vi "GFITS_HdrType2.vi"(10 "keyval":string) -> (1 "type":string, 2 "keyval out":string, 3 "specified":bool)   [LabVIEW 2016]
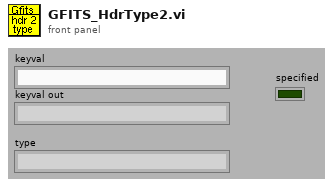
[diagram p1: front panel]
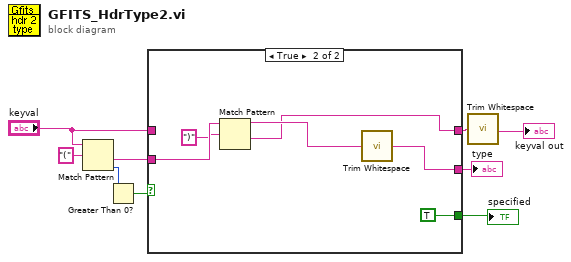
[diagram p0: block diagram]
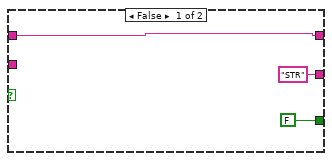
[diagram p2: hidden frame]
diagram:
  n1 = Match Pattern(string="keyval", regular expression="(") -> (after substring=w8:string, offset past match=w7:i32)  [unwired: 3 out]
  n2 = Greater Than 0?(x=w7) -> (x > 0?=w6:bool)
  n3 = case shown="True" w6 {
    tunnel: w8 -> [_ w18]
    tunnel: "keyval" -> [w12 _]
    tunnel: [w12 w14] -> w4
    tunnel: ["STR" ("trimmed string") w16] -> w3
    tunnel: [FALSE ("specified") TRUE ("specified")] -> w1
    frame False {
    }
    frame True {
      n4 = Match Pattern(string=w18, regular expression=")") -> (before substring=w15:string, after substring=w14:string)  [unwired: 3 out]
      n5 = call <vilib>:"Trim Whitespace.vi"("string"=w15) -> ("trimmed string"=w16:string)  [unwired: 1 in]
    }
  }
  "type" <- w3
  "specified" <- w1
  n6 = call <vilib>:"Trim Whitespace.vi"("string"=w4) -> ("trimmed string"=→"keyval out":string)  [unwired: 1 in]
